vi "Tear Down Clock Discipline.vi"(8 "error in (no error)":errorcluster, 11 "RT Data Cluster in":T1={"Timekeeper hdl"="", "clkDisc session"=variant, "Compiled Data"={"SyncMod?"=FALSE, "SyncMod"="", "ConnectionSettings"={"Mode"=enum."Generate sample clock", "pxitrig"=FALSE, "pfi0"=FALSE, "pfi1"=FALSE, "pfi2"=FALSE, "External Pin"=enum."PFI0", "Routes"=[]}, "TimeKeeper"="", "ScanOffset(%)"=0.0, "StartDelay(s)"=0, "Time Ref Settings"={"Time Reference"=enum."GPS", "Priority 1"=0, "Priority 2"=0, "IRIG type"=enum."IRIGB AM", "Terminal"="", "PPSSetTime"=FALSE, "Start Time"=timestamp(0 s since 1904-01-01)}, "FIFO Locations"={"SysTime"=[], "TimeRef"=[], "Status"=[]}}, "OutputsData"=[], "OutputsFIFO"=refnum, "Scan Period"=0, "Timekeeper type"=enum."6683", "SyncMod type"=enum."6683", "SyncMod hdl"=""} {"Compiled Data"."Time Ref Settings"."Priority 2" min=0 max=255; "Compiled Data"."Time Ref Settings"."Priority 1" min=0 max=255}) -> (0 "error out":errorcluster, 3 "RT Data Cluster out":T1={"Timekeeper hdl"="", "clkDisc session"=variant, "Compiled Data"={"SyncMod?"=FALSE, "SyncMod"="", "ConnectionSettings"={"Mode"=enum."Generate sample clock", "pxitrig"=FALSE, "pfi0"=FALSE, "pfi1"=FALSE, "pfi2"=FALSE, "External Pin"=enum."PFI0", "Routes"=[]}, "TimeKeeper"="", "ScanOffset(%)"=0.0, "StartDelay(s)"=0, "Time Ref Settings"={"Time Reference"=enum."GPS", "Priority 1"=0, "Priority 2"=0, "IRIG type"=enum."IRIGB AM", "Terminal"="", "PPSSetTime"=FALSE, "Start Time"=timestamp(0 s since 1904-01-01)}, "FIFO Locations"={"SysTime"=[], "TimeRef"=[], "Status"=[]}}, "OutputsData"=[], "OutputsFIFO"=refnum, "Scan Period"=0, "Timekeeper type"=enum."6683", "SyncMod type"=enum."6683", "SyncMod hdl"=""} {"Compiled Data"."Time Ref Settings"."Priority 2" min=0 max=255; "Compiled Data"."Time Ref Settings"."Priority 1" min=0 max=255})   [LabVIEW 2018, in "Chassis TimeSync Engine.lvlib"]
uses:
  Chassis TimeSync Engine.lvlib
  RT Data Cluster.ctl
  mdevClkDisc.llb/_clkDisc_session.ctl
  Shared/Compiled Data.ctl
  Shared/Connection Settings.ctl
  Shared/Mode.ctl
  Shared/External Pin.ctl
  Shared/Routes.ctl
  Shared/Route.ctl
  Shared/Time Ref Settings.ctl
  Shared/Time Reference.ctl
  Shared/IRIG Type.ctl
  timekeeper type.ctl
  Timekeeper Route Pin.ctl
  Shared/Chassis TimeSync Shared.lvlib
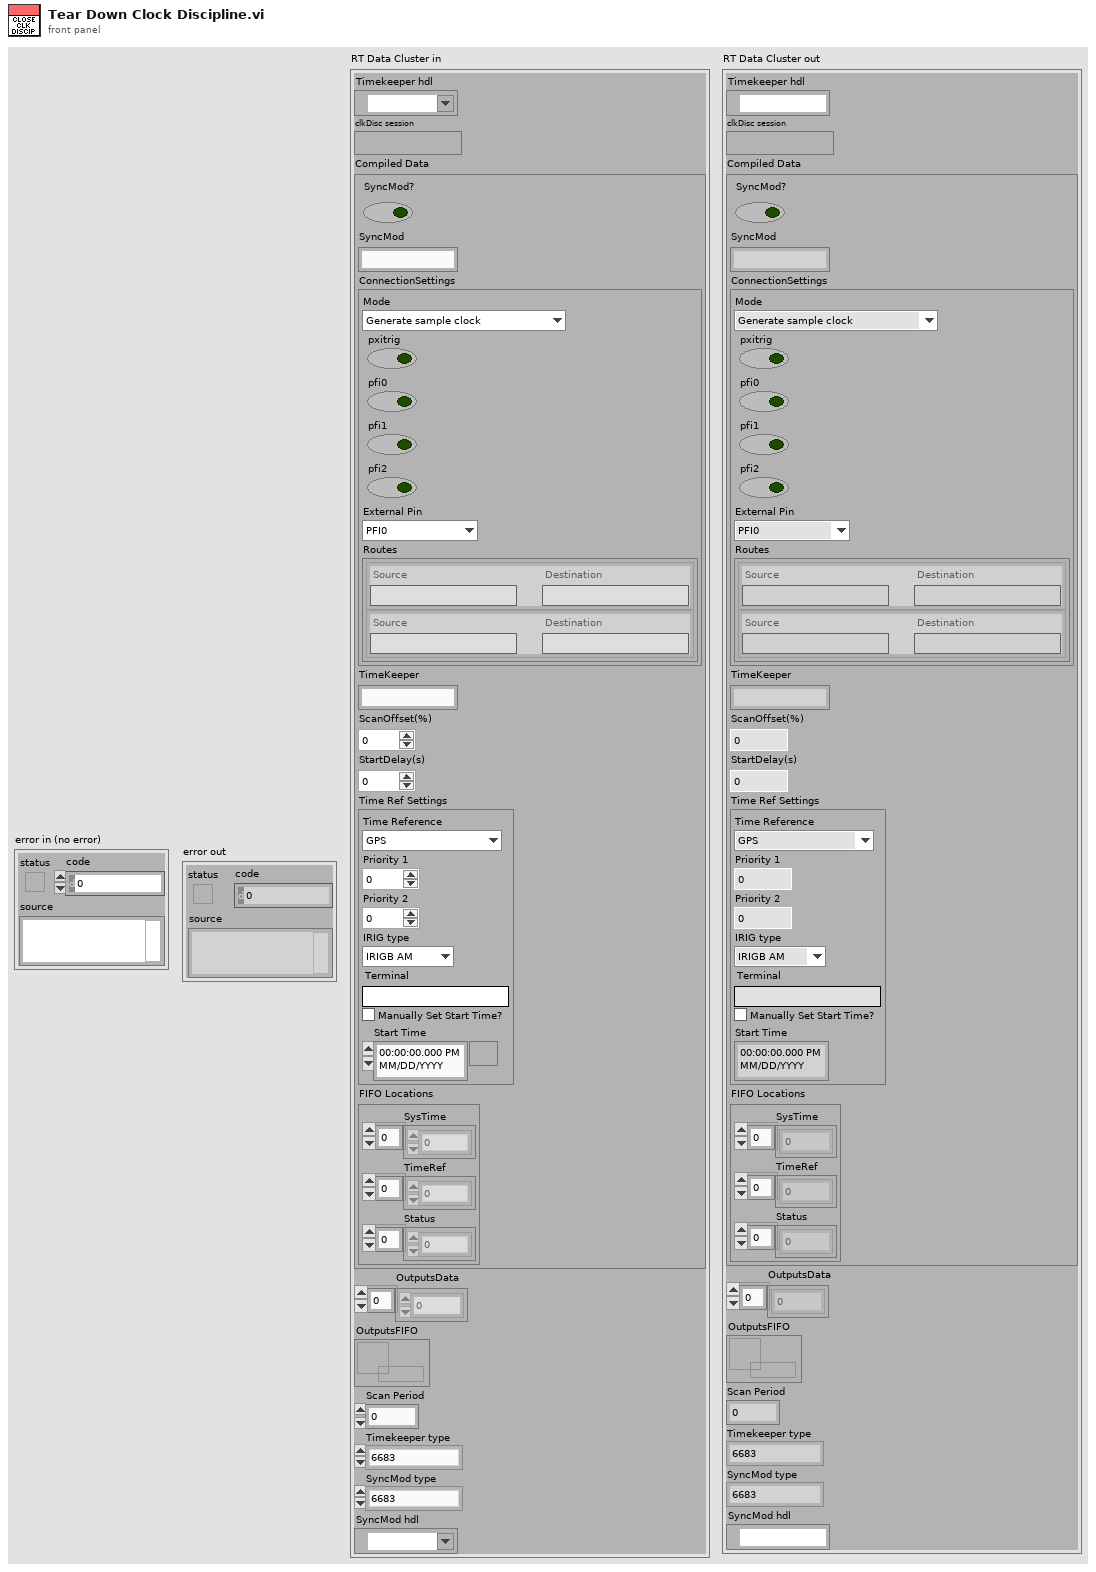
[diagram p1: front panel]
types:
  T1 = typedef "Chassis TimeSync Engine.lvlib/RT Data Cluster.ctl" = cluster{"Timekeeper hdl":refnum<k15>, "clkDisc session":T2, "Compiled Data":T3, "OutputsData":dbl[], "OutputsFIFO":refnum<k33>, "Scan Period":u32, "Timekeeper type":T12, "SyncMod type":T12, "SyncMod hdl":refnum<k15>}
  T2 = typedef "_clkDisc_session.ctl" = variant
  T3 = typedef "Chassis TimeSync Shared.lvlib/Compiled Data.ctl" = cluster{"SyncMod?":bool, "SyncMod":string, "ConnectionSettings":T4, "TimeKeeper":string, "ScanOffset(%)":dbl, "StartDelay(s)":u16, "Time Ref Settings":T9, "FIFO Locations":cluster{"SysTime":i32[], "TimeRef":i32[], "Status":i32[]}}
  T4 = typedef "Chassis TimeSync Shared.lvlib/Connection Settings.ctl" = cluster{"Mode":T5, "pxitrig":bool, "pfi0":bool, "pfi1":bool, "pfi2":bool, "External Pin":T6, "Routes":T7}
  T5 = typedef "Chassis TimeSync Shared.lvlib/Mode.ctl" = enum16{"Generate sample clock", "Route sample clock out of chassis", "Route sample clock into chassis", "Custom routes"}
  T6 = typedef "Chassis TimeSync Shared.lvlib/External Pin.ctl" = enum16{"PFI0", "PFI1", "PFI2"}
  T7 = typedef "Chassis TimeSync Shared.lvlib/Routes.ctl" = T8[]
  T8 = typedef "Chassis TimeSync Shared.lvlib/Route.ctl" = cluster{"Source":string, "Destination":string}
  T9 = typedef "Chassis TimeSync Shared.lvlib/Time Ref Settings.ctl" = cluster{"Time Reference":T10, "Priority 1":i32, "Priority 2":i32, "IRIG type":T11, "Terminal":string, "PPSSetTime":bool, "Start Time":timestamp}
  T10 = typedef "Chassis TimeSync Shared.lvlib/Time Reference.ctl" = enum16{"GPS", "IRIG", "PPS", "1588 Ordinary Clock", "802.1AS", "PXI Chassis Clock", "Free Running (Internal)"}
  T11 = typedef "Chassis TimeSync Shared.lvlib/IRIG Type.ctl" = enum16{"IRIGB DC", "IRIGB AM"}
  T12 = typedef "Chassis TimeSync Engine.lvlib/timekeeper type.ctl" = enum16{"6683", "6683H", "6682", "6682H", "non-timekeeper", "timekeeper"}
  T13 = typedef "Chassis TimeSync Engine.lvlib/Timekeeper Route Pin.ctl" = enum16{"TTL0", "PFI0", "PFI1", "PFI2", "PXI_Clk10", "PXI_Clk10_In", "BoardClk", "ClkOut", "Oscillator"}
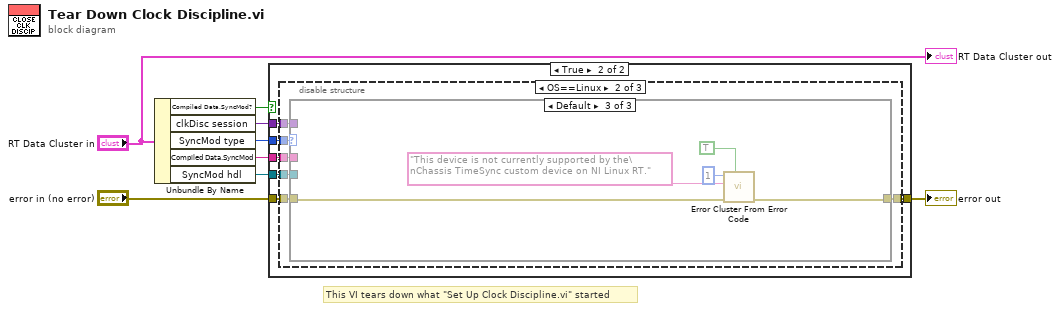
[diagram p0: block diagram]
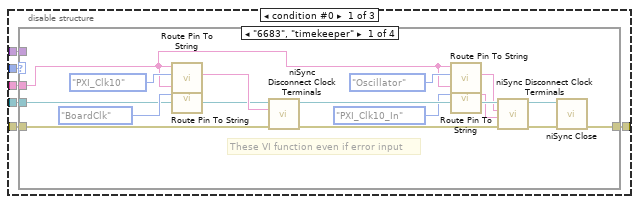
[diagram p3: hidden frame]
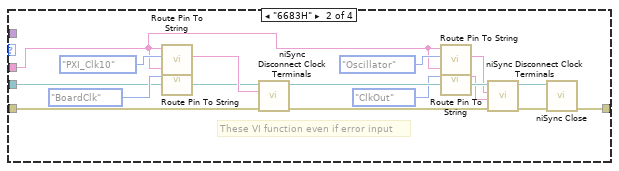
[diagram p4: hidden frame]
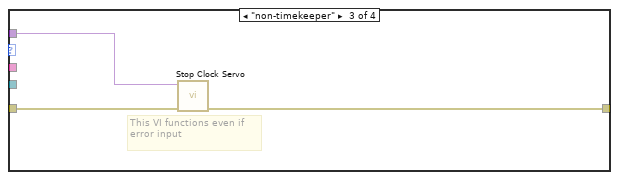
[diagram p5: hidden frame]
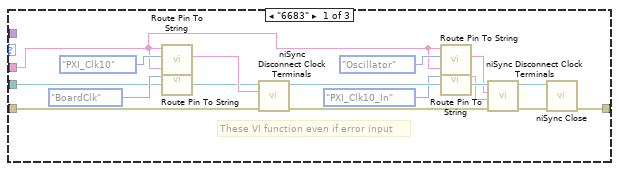
[diagram p7: hidden frame]
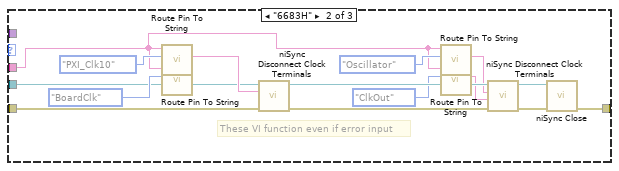
[diagram p8: hidden frame]
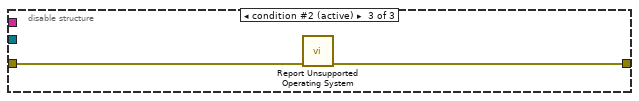
[diagram p9: hidden frame]
diagram:
  # "This VI tears down what \"Set Up Clock Discipline.vi\" started"
  n1 = Unbundle By Name("RT Data Cluster in") -> ("Compiled Data.SyncMod?"=w8:bool, "clkDisc session"=w6:T2, "SyncMod type"=w3:T12, "Compiled Data.SyncMod"=w1:string, "SyncMod hdl"=w2:refnum<k15>)
  n2 = case shown="True" w8 {
    tunnel: "error in (no error)" -> [w9 w15]
    tunnel: [w9 w14] -> w4
    tunnel: w6 -> [_ w13]
    tunnel: w3 -> [_ w12]
    tunnel: w2 -> [_ w10]
    tunnel: w1 -> [_ w11]
    frame False {
    }
    frame True {
      n3 = disable-structure shown="OS==Linux" {
        disable-tunnel: w15 -> [w21 w61 w98]
        disable-tunnel: [w20 w60 w97] -> w14
        disable-tunnel: w13 -> [w19 w59 _]
        disable-tunnel: w12 -> [w18 w58 _]
        disable-tunnel: w11 -> [w17 w57 _]
        disable-tunnel: w10 -> [w16 w56 _]
        frame condition #0 {
          n4 = case shown="\"6683\", \"timekeeper\"" w18 {
            tunnel: w21 -> [w34 w49 w54 w55]
            tunnel: [w33 w48 w53 w55] -> w20
            tunnel: w19 -> [_ _ w52 _]
            tunnel: w17 -> [w24 w39 _ _]
            tunnel: w16 -> [w31 w46 _ _]
            frame "6683", "timekeeper" {
              # "These VI function even if error input"
              n5 = call "Route Pin To String.vi"("Pin"=Timekeeper_Route_Pin."PXI_Clk10", "Module"=w24) -> ("String"=w32:string)  [unwired: 9 in]
              n6 = call "Route Pin To String.vi"("Pin"=Timekeeper_Route_Pin."BoardClk", "Module"=w24) -> ()  [unwired: 9 in, 1 out]
              n7 = call <instrlib>:"niSync Disconnect Clock Terminals.vi"("error in (no error)"=w34, "source terminal"=w32, "instrument handle"=w31) -> ("error out"=w29:errorcluster, "instrument handle out"=w30:refnum<k15>)  [unwired: 7 in]
              n8 = call "Route Pin To String.vi"("Pin"=Timekeeper_Route_Pin."Oscillator", "Module"=w24) -> ("String"=w23:string)  [unwired: 9 in]
              n9 = call "Route Pin To String.vi"("Pin"=Timekeeper_Route_Pin."PXI_Clk10_In", "Module"=w24) -> ("String"=w22:string)  [unwired: 9 in]
              n10 = call <instrlib>:"niSync Disconnect Clock Terminals.vi"("error in (no error)"=w29, "destination terminal"=w22, "source terminal"=w23, "instrument handle"=w30) -> ("error out"=w28:errorcluster, "instrument handle out"=w27:refnum<k15>)  [unwired: 6 in]
              n11 = call <instrlib>:"niSync Close.vi"("error in (no error)"=w28, "instrument handle"=w27) -> ("error out"=w33:errorcluster)  [unwired: 9 in]
            }
            frame "6683H" {
              # "These VI function even if error input"
              n12 = call "Route Pin To String.vi"("Pin"=Timekeeper_Route_Pin."PXI_Clk10", "Module"=w39) -> ("String"=w47:string)  [unwired: 9 in]
              n13 = call "Route Pin To String.vi"("Pin"=Timekeeper_Route_Pin."BoardClk", "Module"=w39) -> ()  [unwired: 9 in, 1 out]
              n14 = call <instrlib>:"niSync Disconnect Clock Terminals.vi"("error in (no error)"=w49, "source terminal"=w47, "instrument handle"=w46) -> ("error out"=w44:errorcluster, "instrument handle out"=w45:refnum<k15>)  [unwired: 7 in]
              n15 = call "Route Pin To String.vi"("Pin"=Timekeeper_Route_Pin."Oscillator", "Module"=w39) -> ("String"=w38:string)  [unwired: 9 in]
              n16 = call "Route Pin To String.vi"("Pin"=Timekeeper_Route_Pin."ClkOut", "Module"=w39) -> ("String"=w37:string)  [unwired: 9 in]
              n17 = call <instrlib>:"niSync Disconnect Clock Terminals.vi"("error in (no error)"=w44, "destination terminal"=w37, "source terminal"=w38, "instrument handle"=w45) -> ("error out"=w43:errorcluster, "instrument handle out"=w42:refnum<k15>)  [unwired: 6 in]
              n18 = call <instrlib>:"niSync Close.vi"("error in (no error)"=w43, "instrument handle"=w42) -> ("error out"=w48:errorcluster)  [unwired: 9 in]
            }
            frame "non-timekeeper" {
              # "This VI functions even if error input"
              n19 = call "Stop Clock Servo.vi"("error (in)"=w54, "clkDisc session (in)"=w52) -> ("error (out)"=w53:errorcluster)  [unwired: 5 in]
            }
            frame "6682", "6682H" {
              # "This would have thrown an error in Set Up Clock Discipline. Pass through error"
            }
          }
        }
        frame condition #1 {
          n20 = case shown="Default" w58 {
            tunnel: w61 -> [w74 w89 w93]
            tunnel: [w73 w88 w92] -> w60
            tunnel: w59 -> [_ _ _]
            tunnel: w57 -> [w64 w79 _]
            tunnel: w56 -> [w71 w86 _]
            frame "6683" {
              # "These VI function even if error input"
              n21 = call "Route Pin To String.vi"("Pin"=Timekeeper_Route_Pin."PXI_Clk10", "Module"=w64) -> ("String"=w72:string)  [unwired: 9 in]
              n22 = call "Route Pin To String.vi"("Pin"=Timekeeper_Route_Pin."BoardClk", "Module"=w64) -> ()  [unwired: 9 in, 1 out]
              n23 = call <instrlib>:"niSync Disconnect Clock Terminals.vi"("error in (no error)"=w74, "source terminal"=w72, "instrument handle"=w71) -> ("error out"=w69:errorcluster, "instrument handle out"=w70:refnum<k15>)  [unwired: 7 in]
              n24 = call "Route Pin To String.vi"("Pin"=Timekeeper_Route_Pin."Oscillator", "Module"=w64) -> ("String"=w63:string)  [unwired: 9 in]
              n25 = call "Route Pin To String.vi"("Pin"=Timekeeper_Route_Pin."PXI_Clk10_In", "Module"=w64) -> ("String"=w62:string)  [unwired: 9 in]
              n26 = call <instrlib>:"niSync Disconnect Clock Terminals.vi"("error in (no error)"=w69, "destination terminal"=w62, "source terminal"=w63, "instrument handle"=w70) -> ("error out"=w68:errorcluster, "instrument handle out"=w67:refnum<k15>)  [unwired: 6 in]
              n27 = call <instrlib>:"niSync Close.vi"("error in (no error)"=w68, "instrument handle"=w67) -> ("error out"=w73:errorcluster)  [unwired: 9 in]
            }
            frame "6683H" {
              # "These VI function even if error input"
              n28 = call "Route Pin To String.vi"("Pin"=Timekeeper_Route_Pin."PXI_Clk10", "Module"=w79) -> ("String"=w87:string)  [unwired: 9 in]
              n29 = call "Route Pin To String.vi"("Pin"=Timekeeper_Route_Pin."BoardClk", "Module"=w79) -> ()  [unwired: 9 in, 1 out]
              n30 = call <instrlib>:"niSync Disconnect Clock Terminals.vi"("error in (no error)"=w89, "source terminal"=w87, "instrument handle"=w86) -> ("error out"=w84:errorcluster, "instrument handle out"=w85:refnum<k15>)  [unwired: 7 in]
              n31 = call "Route Pin To String.vi"("Pin"=Timekeeper_Route_Pin."Oscillator", "Module"=w79) -> ("String"=w78:string)  [unwired: 9 in]
              n32 = call "Route Pin To String.vi"("Pin"=Timekeeper_Route_Pin."ClkOut", "Module"=w79) -> ("String"=w77:string)  [unwired: 9 in]
              n33 = call <instrlib>:"niSync Disconnect Clock Terminals.vi"("error in (no error)"=w84, "destination terminal"=w77, "source terminal"=w78, "instrument handle"=w85) -> ("error out"=w83:errorcluster, "instrument handle out"=w82:refnum<k15>)  [unwired: 6 in]
              n34 = call <instrlib>:"niSync Close.vi"("error in (no error)"=w83, "instrument handle"=w82) -> ("error out"=w88:errorcluster)  [unwired: 9 in]
            }
            frame Default {
              n35 = call <vilib>:"Error Cluster From Error Code.vi"("show call chain? (False)"=TRUE, "error in (no error)"=w93, "error message (\"\")"="This device is not currently supported by the\nChassis TimeSync custom device on NI Linux RT." ("error message (\"\")"), "error code (0)"=1) -> ("error out"=w92:errorcluster)  [unwired: 5 in]
            }
          }
        }
        frame condition #2 (active) {
          n36 = call "Report Unsupported Operating System.vi"("error in (no error)"=w98) -> ("error out"=w97:errorcluster)  [unwired: 10 in]
        }
      }
    }
  }
  "error out" <- w4
  "RT Data Cluster out" <- "RT Data Cluster in"
